vi "BusInOut_input.vi"(8 "error in (no error)":errorcluster, 11 "BusInOut in":refnum<class "BusInOut.lvclass">) -> (0 "error out":errorcluster, 3 "BusInOut out":refnum<class "BusInOut.lvclass">)   [LabVIEW 2011, in "mbed_LVLibrary.lvlib" / "BusInOut.lvclass"]
uses:
  BusInOut.lvclass
  BusInOut.lvclass/BusInOut.ctl
  Transport Mechanisms/mbed/mbed.lvclass
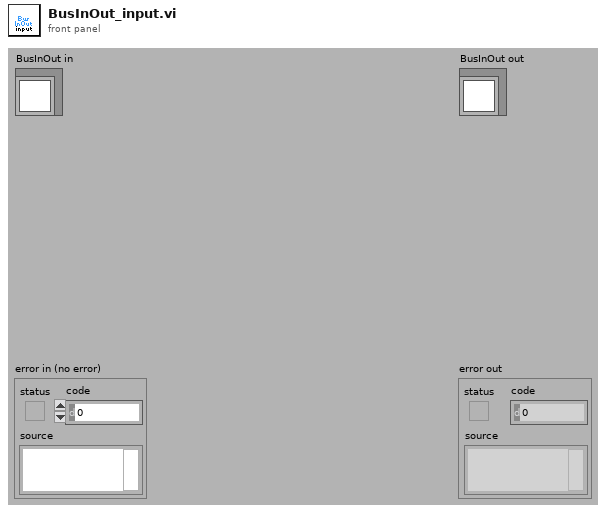
[diagram p1: front panel]
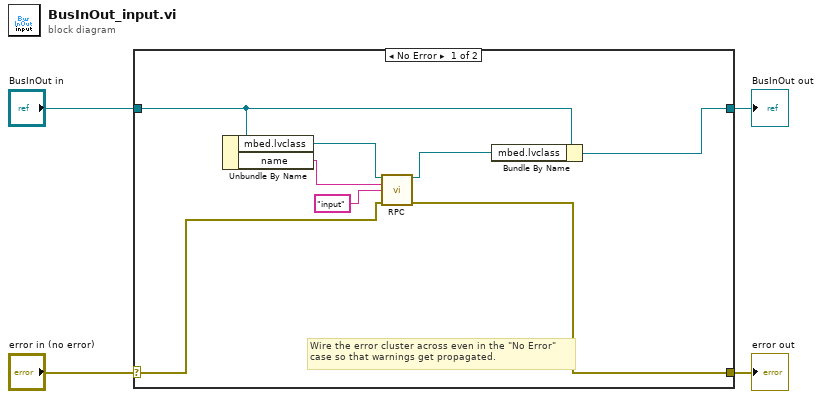
[diagram p0: block diagram]
diagram:
  n1 = case shown="No Error" "error in (no error)" {
    selector: "error in (no error)" -> [w6 w14]
    tunnel: [w5 w14] -> w3
    tunnel: [w11 w13] -> w1
    tunnel: "BusInOut in" -> [w12 w13]
    frame No Error {
      # "Wire the error cluster across even in the \"No Error\"\ncase so that warnings get propagated."
      n2 = Unbundle By Name(w12) -> ("mbed.lvclass"=w10:refnum<class "mbed.lvclass">, "name"=w9:string)
      n3 = call-dynamic "RPC.vi"("mbed in"=w10, "Name"=w9, "method"="input", "error in (no error)"=w6) -> ("mbed out"=w8:refnum<class "mbed.lvclass">, "error out"=w5:errorcluster)  [unwired: 9 in, 1 out]
      n4 = Bundle By Name(cluster=w12, "mbed.lvclass"=w8) -> (w11:refnum<class "BusInOut.lvclass">)
    }
    frame Error {
    }
  }
  "error out" <- w3
  "BusInOut out" <- w1
